vi "PCert-Application-Dir-Database.vi"(8 "error in":errorcluster, 11 "Support Resource Relative Filepath":string) -> (0 "error out":errorcluster, 3 "Support Path":path)   [LabVIEW 2013]
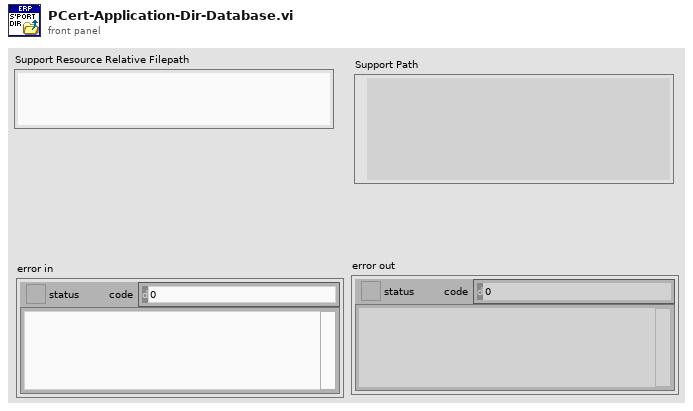
[diagram p1: front panel]
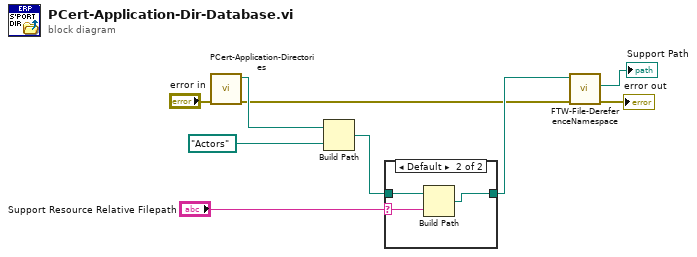
[diagram p0: block diagram]
diagram:
  n1 = call "PCert-Application-Directories.vi"("error in"="error in") -> ("error out"=w4:errorcluster, "Deploy Root"=w6:path)  [unwired: 8 in, 1 out]
  n2 = Build Path(base path=w6, name or relative path=path "Actors") -> (appended path=w8:path)
  n3 = case shown="Default" "Support Resource Relative Filepath" {
    selector: "Support Resource Relative Filepath" -> [_ w11]
    tunnel: [w10 w13] -> w5
    tunnel: w8 -> [w10 w12]
    frame "" {
    }
    frame Default {
      n4 = Build Path(base path=w12, name or relative path=w11) -> (appended path=w13:path)
    }
  }
  n5 = call "FTW-File-DereferenceNamespace.vi"("error in"=w4, "Base Filepath"=w5) -> ("error out"=→"error out":errorcluster, "Actual Filepath"=→"Support Path":path)  [unwired: 8 in]
